vi "ep_Repack Data.vi"(7 "reset? (F)":bool, 8 "error in (no error)":errorcluster, 9 "system info in":refnum<class "EP System Info.lvclass">, 10 "cycles per block":u16, 11 "resampled data":T1) -> (0 "error out":errorcluster, 1 "system info out":refnum<class "EP System Info.lvclass">, 3 "output data blocks":T1[](array[typedef]))   [LabVIEW 2013, in "NI_EP_Power Quality.lvlib"]
uses:
  <vilib>/addons/Electrical Power/PQ/NI_EP_Power Quality.lvlib
  <vilib>/addons/Electrical Power/PQ/Common/Classes/System Info/EP System Info.lvclass
  <vilib>/addons/Electrical Power/PQ/Resampling/Desktop/subVIs/ep_Resampled Data.ctl
  <vilib>/addons/Electrical Power/PQ/Resampling/NI_EP_Resample_Host.lvlib
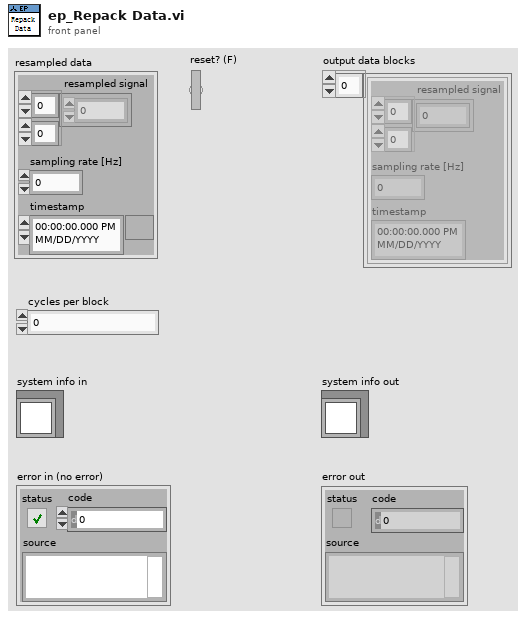
[diagram p1: front panel]
types:
  T1 = typedef "NI_EP_Resample_Host.lvlib/ep_Resampled Data.ctl" = cluster{"resampled signal":dbl[][], "sampling rate [Hz]":dbl, "timestamp":timestamp}
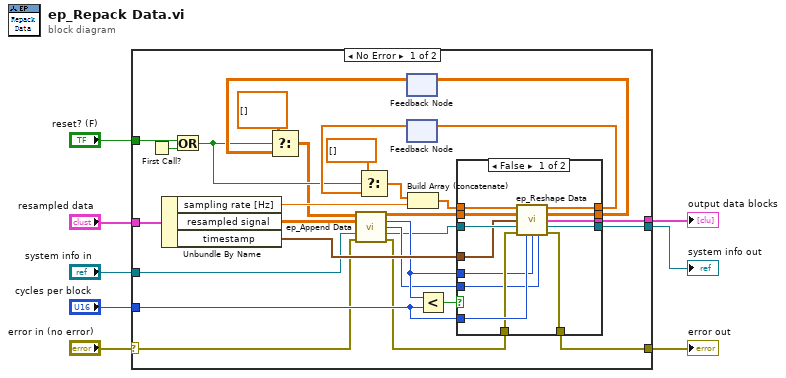
[diagram p0: block diagram]
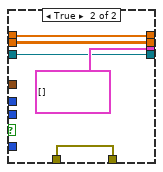
[diagram p2: hidden frame]
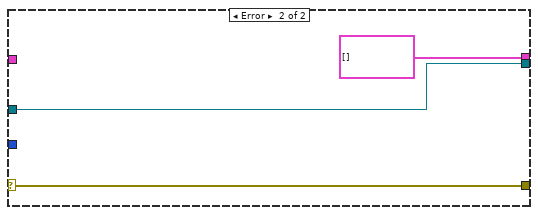
[diagram p3: hidden frame]
diagram:
  n1 = case shown="No Error" "error in (no error)" {
    selector: "error in (no error)" -> [w10 w56]
    tunnel: "cycles per block" -> [w34 _]
    tunnel: [w36 T1[] [] ("output elements")] -> w6
    tunnel: "resampled data" -> [w30 _]
    tunnel: "system info in" -> [w22 w57]
    tunnel: [w15 w57] -> w4
    tunnel: [w31 w56] -> w3
    tunnel: "reset? (F)" -> [w32 _]
    frame No Error {
      n2 = First Call?() -> (First Call?: T/F=w33:bool)
      n3 = Unbundle By Name(w30) -> ("sampling rate [Hz]"=w26:dbl, "resampled signal"=w23:dbl[][], "timestamp"=w24:timestamp)
      n4 = Or(x=w32, y=w33) -> (x .or. y?=w17:bool)
      n5 = feedback #1() -> (w18:dbl[][])  [unwired: 1 in]
      n6 = Select(t=dbl[][] [] ("appended signal"), s=w17, f=w18) -> (s? t:f=w16:dbl[][])
      n7 = call <vilib>:"ep_Append Data.vi"("history data"=w16, "current data"=w23, "system info in"=w22, "error in (no error)"=w10) -> ("appended signal"=w21:dbl[][], "total cycles"=w14:i32, "total size"=w13:i32, "system info out"=w11:refnum<class "EP System Info.lvclass">, "error out"=w9:errorcluster)  [unwired: 7 in]
      n8 = feedback #2() -> (w29:dbl[])  [unwired: 1 in]
      n9 = Select(t=dbl[] [], s=w17, f=w29) -> (s? t:f=w28:dbl[])
      n10 = Build Array (concatenate)(w28, w26) -> (w12:dbl[])
      n11 = Less?(x=w14, y=w34) -> (x < y?=w35:bool)
      n12 = case shown="False" w35 {
        tunnel: [w40 T1[] [] ("output elements")] -> w36
        tunnel: w34 -> [w45 _]
        tunnel: w9 -> [w44 w53]
        tunnel: [w43 w53] -> w31
        tunnel: w12 -> [w49 w52]
        tunnel: [w41 w52] -> w25
        tunnel: w24 -> [w46 _]
        tunnel: w21 -> [w48 w51]
        tunnel: [w42 w51] -> w20
        tunnel: w11 -> [w47 w50]
        tunnel: [w39 w50] -> w15
        tunnel: w14 -> [w38 _]
        tunnel: w13 -> [w37 _]
        frame False {
          n13 = call <vilib>:"ep_Reshape Data.vi"("sampling rate in"=w49, "appended signal"=w48, "timestamp"=w46, "system info in"=w47, "error in (no error)"=w44, "cycles per block"=w45, "input cycles"=w38, "input size"=w37) -> ("sampling rate out"=w41:dbl[], "remained signal"=w42:dbl[][], "output data blocks"=w40:T1[], "system info out"=w39:refnum<class "EP System Info.lvclass">, "error out"=w43:errorcluster)  [unwired: 3 in]
        }
        frame True {
        }
      }
      n14 = feedback-in #1(w20) -> ()
      n15 = feedback-in #2(w25) -> ()
    }
    frame Error {
    }
  }
  "output data blocks" <- w6
  "system info out" <- w4
  "error out" <- w3
